vi "SV_Process.vi"(0 "Process Data":T2={"Write URLs"={"URLs"=[]}, "Read URLs"={"URLs"=[]}, "Write SV FIFO"="", "Read SV FIFO"="", "Status SV FIFO"="", "Status Notifier"="", "Update Rate"=10}) -> (10 "error out":errorcluster)   [LabVIEW 2020, in "Shared Variable Interface.lvlib"]
uses:
  Shared Variable Interface.lvlib
  Shared DataTypes/URLs.ctl
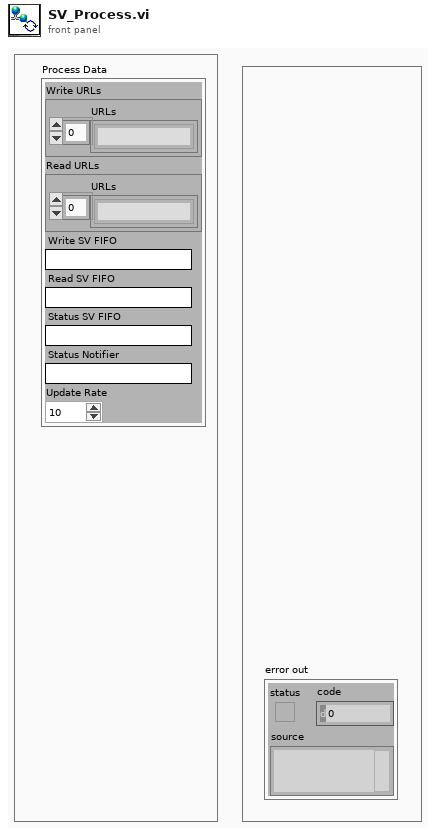
[diagram p1: front panel]
types:
  T1 = typedef "URLs.ctl" = cluster{"URLs":string[]}
  T2 = cluster{"Write URLs":T1, "Read URLs":T1, "Write SV FIFO":string, "Read SV FIFO":string, "Status SV FIFO":string, "Status Notifier":string, "Update Rate":u32}
  T3 = typedef "Shared Variable Interface.lvlib/SV Process Configuration.ctl" = cluster{"Status notifier":refnum<notifier>, "Write FIFO ref":refnum<k33>, "Read FIFO ref":refnum<k33>, "Status FIFO ref":refnum<k33>, "Update Rate":u32, "Write Refs by Type":cluster{"DBL Write":refnum<k21>[], "Bool Write":refnum<k21>[], "DBLIndex":i32[], "BoolIndex":i32[]}, "Read Refs by Type":cluster{"DBL Read":refnum<k21>[], "Bool Read":refnum<k21>[], "DBLIndex":i32[], "BoolIndex":i32[]}, "WriteSize":i32, "ReadSize":i32}
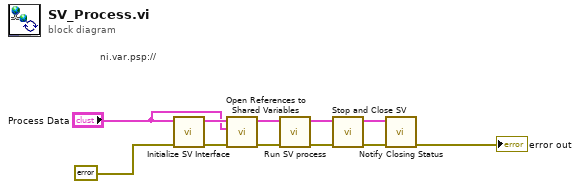
[diagram p0: block diagram]
diagram:
  # "ni.var.psp://"
  n1 = call "Initialize SV Interface.vi"("error in (no error)"=errorcluster {"status"=FALSE, "code"=0, "source"=""}, "Process Data"="Process Data") -> ("error out"=w11:errorcluster, "SV Data"=w6:T3)  [unwired: 8 in]
  n2 = call "Open References to Shared Variables.vi"("error in (no error)"=w11, "Process Data"="Process Data", "SV Data"=w6) -> ("error out"=w10:errorcluster, "SV Data"=w5:T3)  [unwired: 7 in]
  n3 = call "Run SV process.vi"("error in (no error)"=w10, "SV Data"=w5) -> ("error out"=w7:errorcluster, "SV Data"=w4:T3)  [unwired: 8 in]
  n4 = call "Stop and Close SV.vi"("error in (no error)"=w7, "SV Data"=w4) -> ("error out"=w9:errorcluster, "SV Data"=w3:T3)  [unwired: 8 in]
  n5 = call "Notify Closing Status.vi"("error in (no error)"=w9, "SV Data"=w3) -> ("error out"=→"error out":errorcluster)  [unwired: 9 in]
